vi "VI Server Control N2 Com.vi"(1 "command text in":string[](array[string]), 2 "option":T3) -> (0 "Command text out":string[][](array[string]))   [LabVIEW 2020]
uses:
  Ctl/option.ctl
  VI Server Control N2.ctl
  condition.ctl
panel:
  in  "VI Server Control N2":T1={"VI name"="", "Control"=[], "Value"=[], "Boolean?"=[], "Wait Option"=enum."Wait Until", "wait (sec)"=10.0, "Control to End"="", "finish boolean?"=enum."boolean", "Condition"=enum."within xxx% of target value", "Target Value"=0.0, "xxx%"=0.0, "update every (s)"=120.0, "Timeout (sec)"=10000.0} {"Boolean?" min=0.0 max=1.0 step=1.0 format="%#_1g"}
  in  "cancel":bool
  in  "enter":bool
  # "Value of Control\n(if control is boolean type\n1 for \"ON\" and,0 for \"OFF\")"
  # "Is this control Boolean?\n(Yes: 1,  No: 0)"
  # "Name of  Control"
  # "0"
  # "1"
  # "2"
  # "3"
  # "4"
  # "5"
  # "6"
  # "7"
  # "8"
  # "9"
  # "1."
  # "Purely wait for"
  # "seconds"
  # "2."
  # "Control / Indicator Name"
  # "which is"
  # "Finish if"
  # "meets the following conditions"
  # "(check and update every"
  # "seconds)"
  # "3. Timeout"
  # "Wait until the following condition meets."
  # "Do not wait and move on to the next line in sequence."
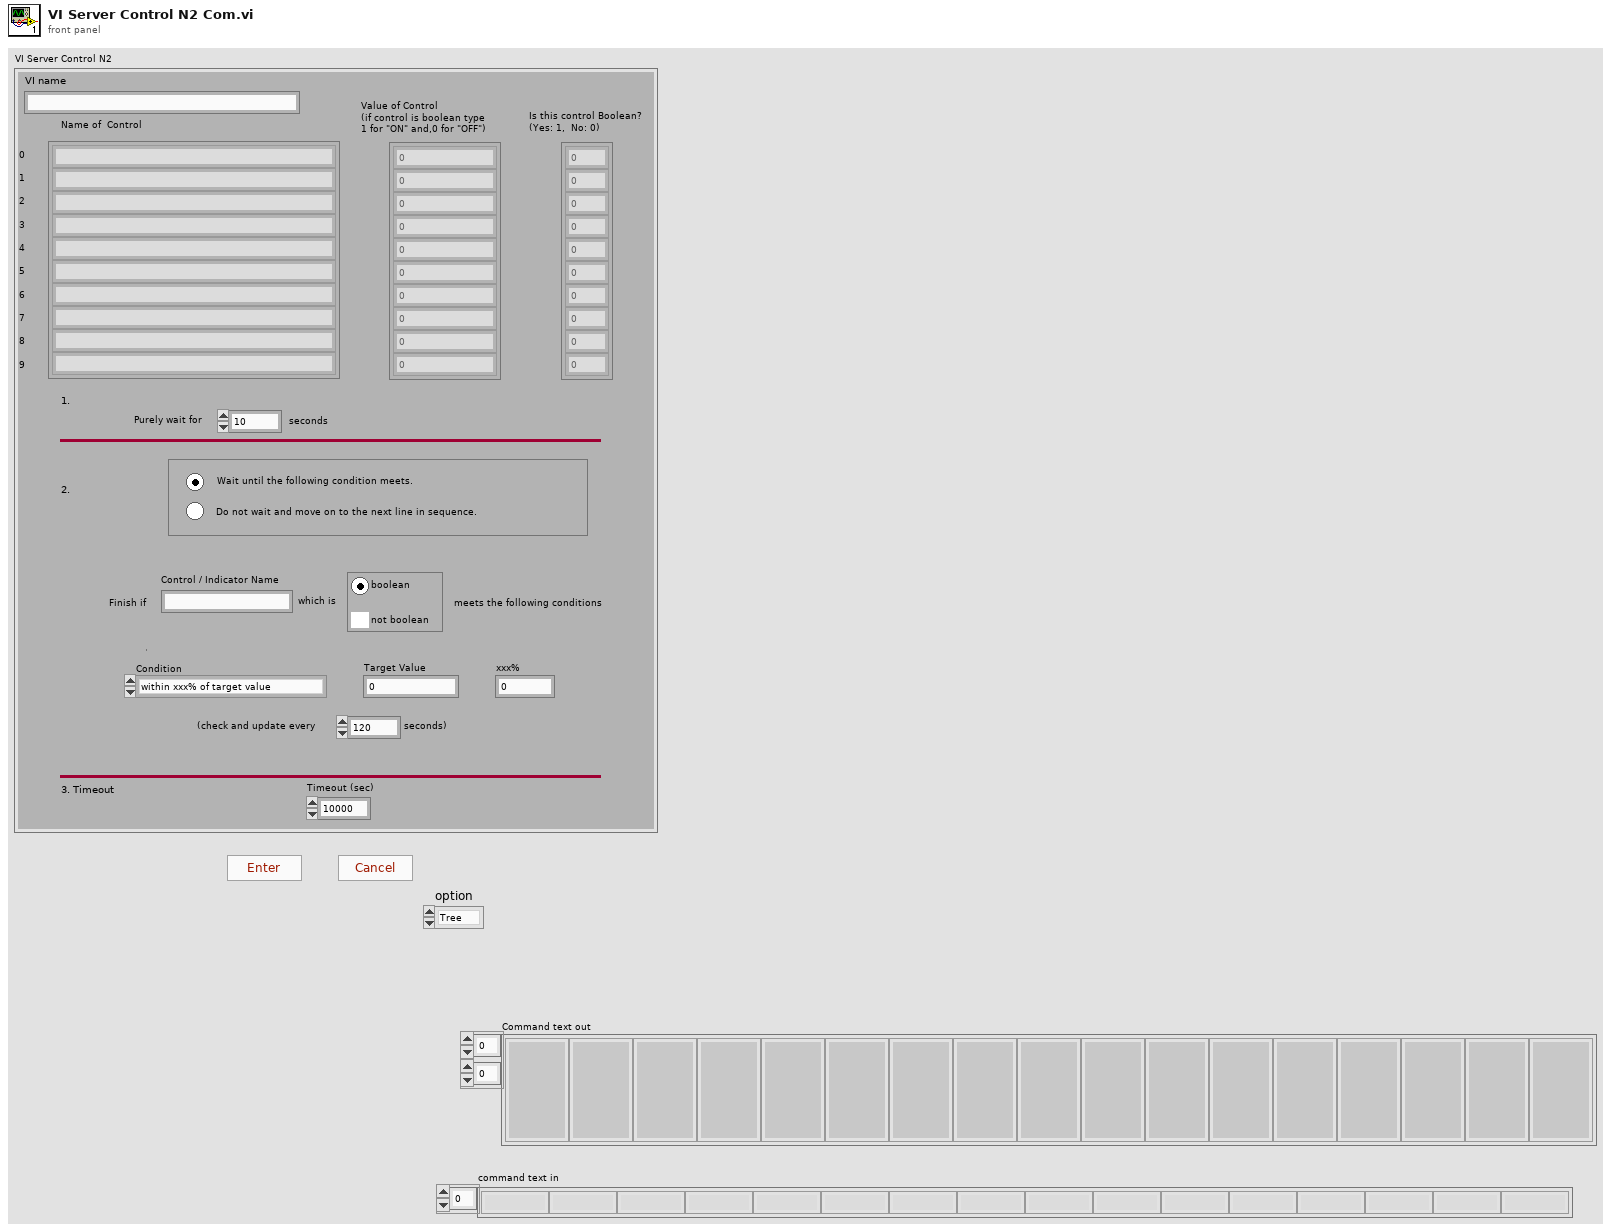
[diagram p1: front panel]
types:
  T1 = typedef "VI Server Control N2.ctl" = cluster{"VI name":string, "Control":string[], "Value":dbl[], "Boolean?":dbl[], "Wait Option":enum32{"Wait Until", "Do Not Wait"}, "wait (sec)":dbl, "Control to End":string, "finish boolean?":enum32{"boolean", "not boolean"}, "Condition":T2, "Target Value":dbl, "xxx%":dbl, "update every (s)":dbl, "Timeout (sec)":dbl}
  T2 = typedef "condition.ctl" = enum16{"within xxx% of target value", "<= target value", ">= target value", "= target value", "Boolean ON", "Boolean OFF"}
  T3 = typedef "option.ctl" = enum16{"Tree", "List"}
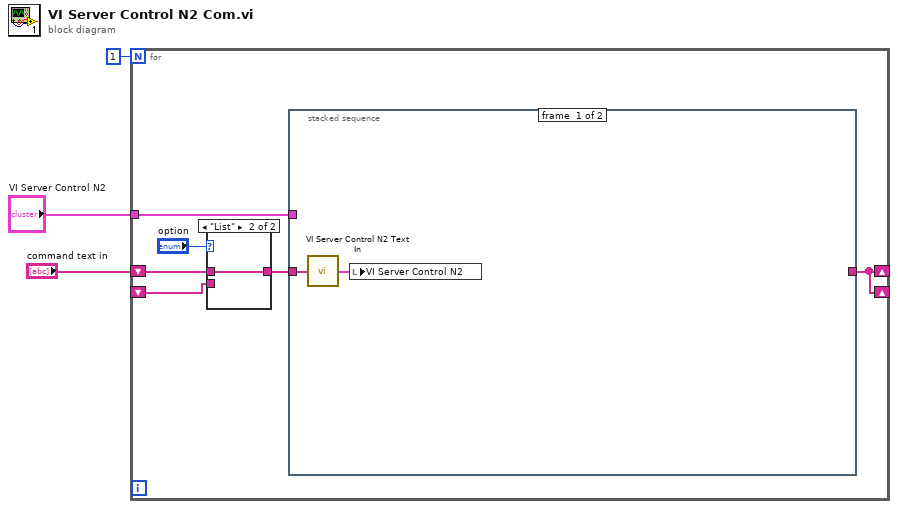
[diagram p0: block diagram]
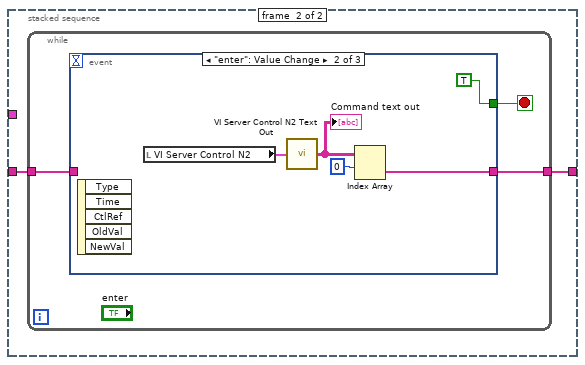
[diagram p3: hidden frame]
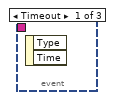
[diagram p4: hidden frame]
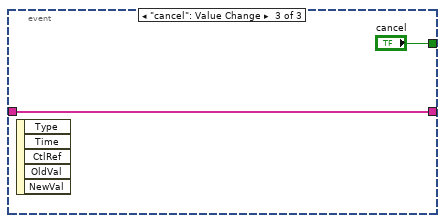
[diagram p5: hidden frame]
diagram:
  n1 = for {
    N: 1 -> [_]
    shift-right: [w4] -> _
    shift-left: _ -> [w8]
    shift-right: [w4] -> _
    shift-left: "command text in" -> [w7]
    tunnel: "VI Server Control N2" -> [w5]
    n2 = case shown="\"List\"" "option" {
      tunnel: [w10 w11] -> w9
      tunnel: w8 -> [w10 _]
      tunnel: w7 -> [_ w11]
      frame "Tree", Default {
      }
      frame "List" {
      }
    }
    n3 = stacked-sequence {
      tunnel: [_ w15] -> w4
      tunnel: w9 -> [w13 w14]
      tunnel: w5 -> [_ _]
      frame #0 {
        n4 = call "VI Server Control N2 Text In.vi"("command text in"=w13) -> ("VI Server Control N2"=w12:T1)
        n5 = local write "VI Server Control N2"(w12) -> ()
      }
      frame #1 {
        n6 = while {
          tunnel: [w17] -> w15
          tunnel: w14 -> [w16]
          stop <- w18 stop-if-true
          n7 = event shown="[1] \"enter\": Value Change" {
            selector: _ -> [_ _ _]
            dyn-events: _ -> [_ _ _]
            timeout: _ -> [_ _ _]
            tunnel: [_ TRUE "cancel"] -> w18
            tunnel: [_ w23 w24] -> w17
            tunnel: w16 -> [_ _ w24]
            event Timeout {
              n8 = event-data() -> ()  [unwired: 1 in, 2 out]
            }
            event "enter": Value Change {
              n9 = event-data() -> ()  [unwired: 1 in, 5 out]
              n10 = local read "VI Server Control N2"() -> (w20:T1)
              n11 = call "VI Server Control N2 Text Out.vi"("VI Server Control N2"=w20) -> ("Command text"=w19:string[][])
              "Command text out" <- w19
              n12 = Index Array(array=w19, index (row)=0 ("disabled index (col)")) -> (element=w23:string[])  [unwired: 1 in]
            }
            event "cancel": Value Change {
              n13 = event-data() -> ()  [unwired: 1 in, 5 out]
            }
          }
        }
      }
    }
  }
